vi "map_history_global.vi"() -> ()   [LabVIEW 2015]
uses:
  map_data.ctl
  <vilib>/Utility/miscctls.llb/LVOffsetAndMultiplierTypeDef.ctl
panel:
  in  "saved_map_data":T3
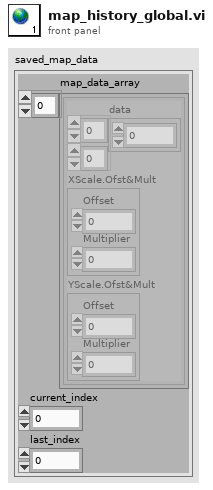
[diagram p1: front panel]
types:
  T1 = typedef "map_data.ctl" = cluster{"data":dbl[][], "XScale.Ofst&Mult":T2, "YScale.Ofst&Mult":T2}
  T2 = typedef "LVOffsetAndMultiplierTypeDef.ctl" = cluster{"Offset":dbl, "Multiplier":dbl}
  T3 = cluster{"map_data_array":T1[], "current_index":i32, "last_index":i32}
diagram:
